vi "Lookup Channels by Meta Values.vi"(8 "error in (no error)":errorcluster, 9 "Meta Values":string[](array[string]), 10 "Meta Name":string, 11 "Group in":refnum<class "Group.lvclass">) -> (0 "error out":errorcluster, 2 "Channels":refnum<class "Channel.lvclass">[](array[class]), 3 "Group out":refnum<class "Group.lvclass">, 5 "Indices":i32[](array[numeric]))   [LabVIEW 2020, in "VolatusConfig.lvlib" / "Group.lvclass"]
uses:
  Group.lvclass
  C:/dev/lv20CE/relink/lv-volatus/VolatusConfig/VolatusConfigElement/VolatusConfigElement.lvclass
  Channel/Channel.lvclass
  VolatusConfigElement/VolatusConfigElement.lvclass/VolatusConfigElement.ctl
  VolatusConfigElement/Element.vi
  VolatusConfigElement/VolatusConfigElement.lvclass
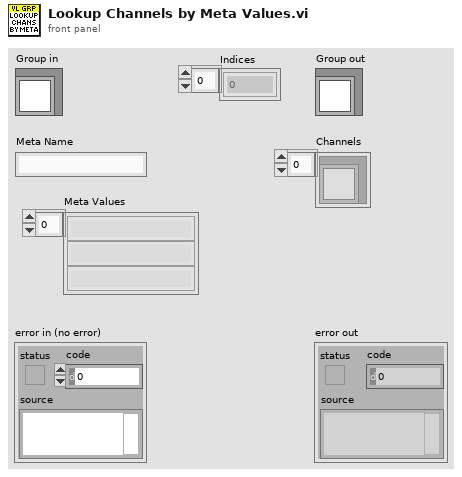
[diagram p1: front panel]
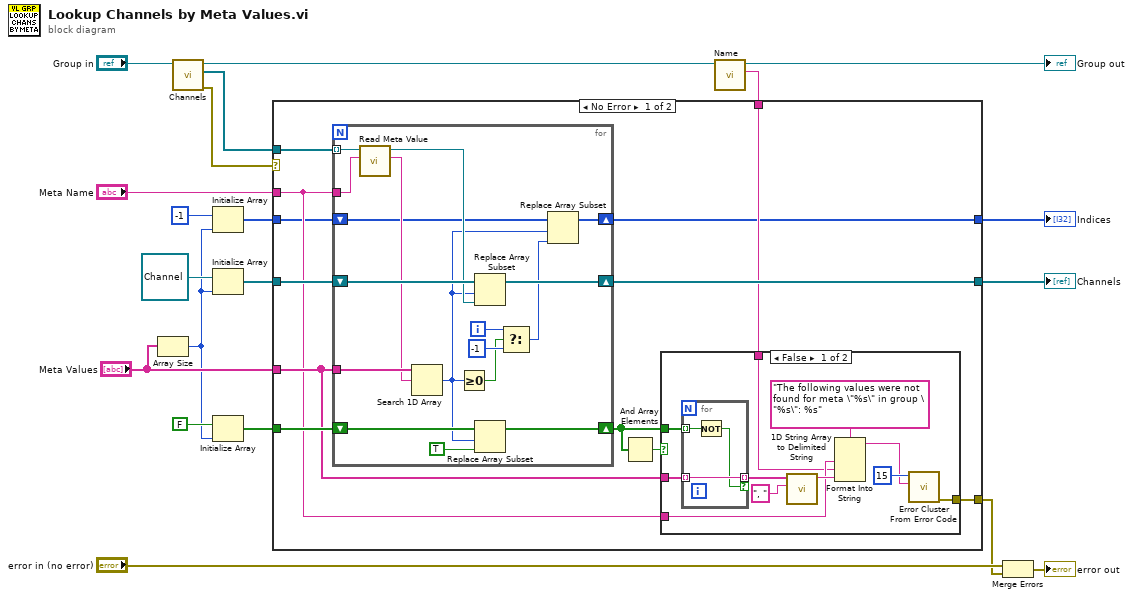
[diagram p0: block diagram]
diagram:
  n1 = Array Size(array="Meta Values") -> (size(s)=w2:i32)
  n2 = call "Channels.vi"("Group in"="Group in") -> ("error out"=w14:errorcluster, "Channels"=w15:refnum<class "Channel.lvclass">[], "Group out"=w12:refnum<class "Group.lvclass">)  [unwired: 8 in]
  n3 = Initialize Array(-1, w2) -> (w1:i32[])
  n4 = Initialize Array(refnum<class "Channel.lvclass"> refnum ("Config Element in"), w2) -> (w9:refnum<class "Channel.lvclass">[])
  n5 = Initialize Array(FALSE, w2) -> (w10:bool[])
  n6 = call "Name.vi"("VolatusConfigElement in"=w12) -> ("Name"=w5:string, "VolatusConfigElement out"=→"Group out":refnum<class "Group.lvclass">)  [unwired: 8 in, 1 out]
  n7 = case shown="No Error" w14 {
    selector: w14 -> [_ w64]
    tunnel: w9 -> [w32 _]
    tunnel: w15 -> [w31 _]
    tunnel: "Meta Values" -> [w26 _]
    tunnel: "Meta Name" -> [w25 _]
    tunnel: [w30 _] -> w8
    tunnel: w10 -> [w29 _]
    tunnel: [w24 w64] -> w4
    tunnel: [w21 _] -> w11
    tunnel: w5 -> [w23 _]
    tunnel: w1 -> [w22 _]
    frame No Error {
      n8 = for {
        shift-right: [w40] -> w30
        shift-left: w32 -> [w46]
        tunnel: w31 -> [w48] mode=indexing
        tunnel: w26 -> [w49]
        tunnel: w25 -> [w47]
        shift-right: [w41] -> w27
        shift-left: w29 -> [w43]
        shift-right: [w33] -> w21
        shift-left: w22 -> [w36]
        i -> [w39]
        n9 = call "Read Meta Value.vi"("Meta Name"=w47, "VolatusConfigElement in"=w48) -> ("Meta Value"=w44:string, "VolatusConfigElement out"=w45:refnum<class "Channel.lvclass">)  [unwired: 7 in, 1 out]
        n10 = Search 1D Array(1D array=w49, element=w44) -> (index of element=w35:i32)  [unwired: 1 in]
        n11 = Greater Or Equal To 0?(x=w35) -> (x >= 0?=w37:bool)
        n12 = Replace Array Subset(array=w46, new element=w45, index=w35) -> (w40:refnum<class "Channel.lvclass">[])
        n13 = Replace Array Subset(array=w43, new element=TRUE ("new element/subarray"), index=w35) -> (w41:bool[])
        n14 = Select(t=w39, s=w37, f=-1) -> (s? t:f=w34:i32)
        n15 = Replace Array Subset(array=w36, new element=w34, index=w35) -> (w33:i32[])
      }
      n16 = And Array Elements(Boolean array=w27) -> (logical AND=w28:bool)
      n17 = case shown="False" w28 {
        tunnel: w27 -> [w60 _]
        tunnel: w26 -> [w59 _]
        tunnel: w25 -> [w51 _]
        tunnel: [w52 _] -> w24
        tunnel: w23 -> [w50 _]
        frame False {
          n18 = for {
            tunnel: w60 -> [w63] mode=indexing
            tunnel: w59 -> [w62] mode=indexing
            tunnel: [w62] -> w58 mode=indexing if=w61
            n19 = Not(x=w63) -> (.not. x?=w61:bool)
          }
          n20 = call <vilib>:"1D String Array to Delimited String.vi"("delimiter"=", ", "string array"=w58) -> ("delimited string"=w56:string)  [unwired: 9 in]
          n21 = Format Into String(format string="The following values were not found for meta \"%s\" in group \"%s\": %s", w51, w50, w56) -> (resulting string=w53:string)  [unwired: 2 in, 1 out]
          n22 = call <vilib>:"Error Cluster From Error Code.vi"("error message (\"\")"=w53, "error code (0)"=15) -> ("error out"=w52:errorcluster)  [unwired: 7 in]
        }
        frame True {
          # "All values were found."
        }
      }
    }
    frame Error {
    }
  }
  "Indices" <- w11
  "Channels" <- w8
  n23 = Merge Errors("error in (no error)", w4) -> (→"error out":errorcluster)
